vi "Utilities_Calculate text position from top.vi"(5 "Line Count":i32=4, 6 "Line Index":i32, 7 "Line Height":i32=5, 8 "Error":errorcluster, 10 "Starting Offset":i32=7, 11 "Field Total Height":i32=24) -> (0 "Error Out":errorcluster, 3 "Text Positn From Top Out":i32)   [LabVIEW 2014]
doc: "Calculates the top position of a line from the inputs"
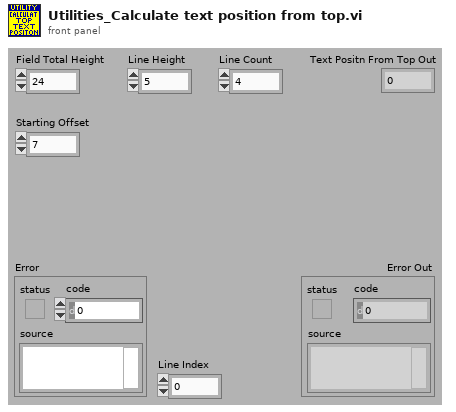
[diagram p1: front panel]
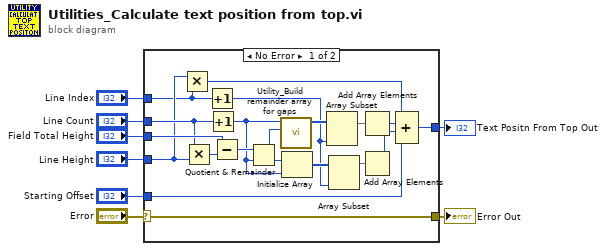
[diagram p0: block diagram]
diagram:
  n1 = case shown="No Error" "Error" {
    selector: "Error" -> [w17 w29]
    tunnel: "Line Count" -> [w20 _]
    tunnel: "Line Height" -> [w19 _]
    tunnel: "Field Total Height" -> [w26 _]
    tunnel: "Starting Offset" -> [w28 _]
    tunnel: [w27 _] -> w4
    tunnel: [w17 w29] -> w3
    tunnel: "Line Index" -> [w18 _]
    frame No Error {
      n2 = Multiply(x=w19, y=w18) -> (x*y=w14:i32)
      n3 = Multiply(x=w20, y=w19) -> (x*y=w24:i32)
      n4 = Increment(x=w18) -> (x+1=w11:i32)
      n5 = Increment(x=w20) -> (x+1=w21:i32)
      n6 = Subtract(x=w26, y=w24) -> (x-y=w25:i32)
      n7 = Quotient & Remainder(x=w25, y=w21) -> (x-y*floor(x/y)=w23:i32, floor(x/y)=w22:i32)
      n8 = call "Utility_Build remainder array for gaps.vi"("Remainder"=w23, "Gap Count"=w21) -> ("Extra gap array"=w13:i16[])  [unwired: 9 in]
      n9 = Initialize Array(w22, w21) -> (w12:i32[])
      n10 = Array Subset(array=w13, length=w11) -> (w10:i16[])  [unwired: 1 in]
      n11 = Array Subset(array=w12, length=w11) -> (w9:i32[])  [unwired: 1 in]
      n12 = Add Array Elements(numeric array=w10) -> (sum=w15:i16)
      n13 = Add Array Elements(numeric array=w9) -> (sum=w16:i32)
      n14 = Compound Arithmetic op=ADD(w14, w15, w16, w28) -> (w27:i32)
    }
    frame Error {
    }
  }
  "Text Positn From Top Out" <- w4
  "Error Out" <- w3
